vi "Where to Fall.vi"(10 "indices in":T1, 11 "Picture in":refnum<class "Picture.lvclass">) -> (1 "indices out":T1, 3 "Picture out":refnum<class "Picture.lvclass">, 5 "nowhere?":bool)   [LabVIEW 2018]
uses:
  Coords.ctl
  Picture.lvclass
  Picture.lvclass/Picture.ctl
  Accessors/Read BG color.vi
  Accessors/Read Pixel.vi
  Accessors/Read Size.vi
  Accessors/Get Pixels Below.vi
panel:
  out "x-y":dbl
  out "Free Pixels":cluster{"Weight":dbl, "indices":T1}[](array[cluster])
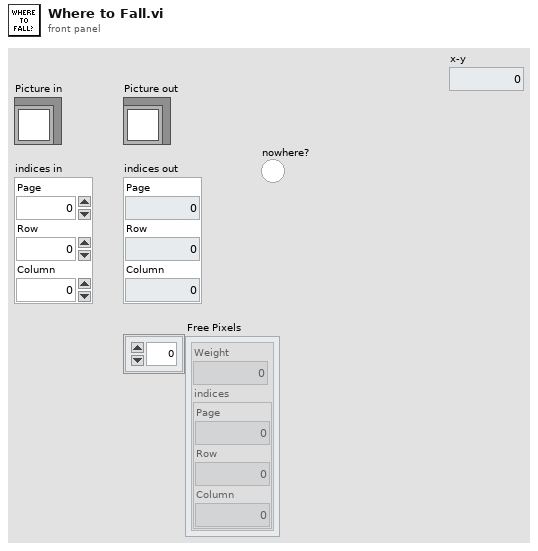
[diagram p1: front panel]
types:
  T1 = typedef "Coords.ctl" = cluster{"Page":i32, "Row":i32, "Column":i32}
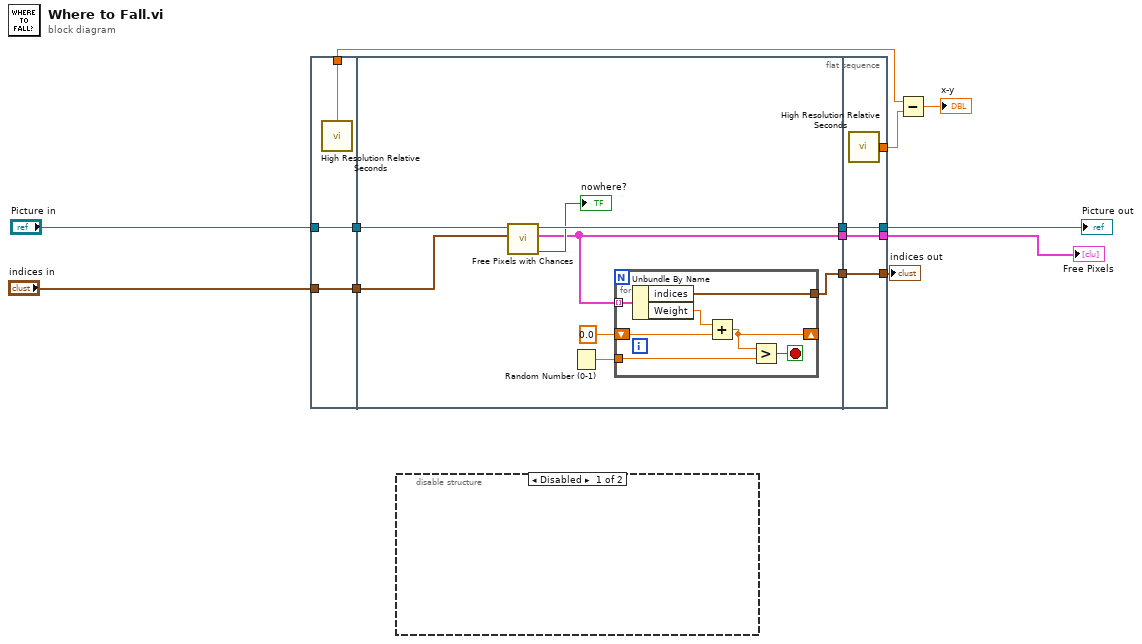
[diagram p0: block diagram]
diagram:
  n1 = flat-sequence {
    tunnel: "Picture in" -> [w15]
    tunnel: "indices in" -> [w16]
    tunnel: [w16] -> w8
    tunnel: [w15] -> w7
    tunnel: [w14] -> w2
    tunnel: w8 -> [w23]
    tunnel: w7 -> [w22]
    tunnel: [w17] -> w6
    tunnel: [w18] -> w5
    tunnel: [w24] -> w4
    tunnel: [w33] -> w11
    tunnel: [w34] -> w12
    tunnel: [w35] -> w13
    tunnel: w6 -> [w35]
    tunnel: w5 -> [w34]
    tunnel: w4 -> [w33]
    tunnel: [w32] -> w3
    frame #0 {
      n2 = call <vilib>:"High Resolution Relative Seconds.vi"() -> ("relative seconds"=w14:dbl)
    }
    frame #1 {
      n3 = call "Free Pixels with Chances.vi"("indices"=w23, "Picture in"=w22) -> ("Empty?"=→"nowhere?":bool, "Free Pixels"=w18:cluster{"Weight":dbl, "indices":T1}[], "Picture out"=w24:refnum<class "Picture.lvclass">)  [unwired: 7 in]
      n4 = Random Number (0-1)() -> (number: 0 to 1=w19:dbl)
      n5 = for {
        tunnel: w18 -> [w31] mode=indexing
        shift-right: [w28] -> _
        shift-left: 0.0 -> [w30]
        tunnel: w19 -> [w29]
        tunnel: [w27] -> w17
        stop <- w25 stop-if-true
        n6 = Unbundle By Name(w31) -> ("indices"=w27:T1, "Weight"=w26:dbl)
        n7 = Add(x=w26, y=w30) -> (x+y=w28:dbl)
        n8 = Greater?(x=w28, y=w29) -> (0:w25:bool)
      }
    }
    frame #2 {
      n9 = call <vilib>:"High Resolution Relative Seconds.vi"() -> ("relative seconds"=w32:dbl)
    }
  }
  n10 = disable-structure shown="Disabled" {
    frame Disabled {
    }
    frame Enabled {
    }
  }
  n11 = Subtract(x=w2, y=w3) -> (x-y=→"x-y":dbl)
  "indices out" <- w13
  "Free Pixels" <- w12
  "Picture out" <- w11
